vi "working.vi"() -> ()   [LabVIEW 2017]
uses:
  <vilib>/myRIO/Instrument Drivers/Onboard IO/DIO/typedefs/DIO Reference.ctl
  <vilib>/myRIO/Common/Instrument Driver Framework/Utilities/typedefs/myRIO Generic Hardware Reference.ctl
  <vilib>/myRIO/Common/Instrument Driver Framework/Utilities/typedefs/Hardware Version Enum.ctl
  <vilib>/myRIO/Common/Instrument Driver Framework/Utilities/typedefs/myRIO v1.0 Reference.ctl
  <vilib>/myRIO/Common/Instrument Driver Framework/Utilities/typedefs/Generic FPGA Reference.ctl
  <vilib>/myRIO/Common/Instrument Driver Framework/myRIO v1.0/DIO/typedefs/DIO Channels List.ctl
  <vilib>/myRIO/Common/Instrument Driver Framework/myRIO v1.0/DIO/typedefs/DIO Channels Enum.ctl
  <vilib>/userdefined/High Color/nirio_resource_hc.ctl
  <vilib>/myRIO/Common/Instrument Driver Framework/Utilities/vis/Is FPGA Ref Available.vi
  <vilib>/myRIO/Common/Instrument Driver Framework/myRIO v1.0/DIO/vis/myRIO v1.1 Open DIO.vi
  <vilib>/myRIO/Instrument Drivers/Onboard IO/DIO/vis/Write.vi
  <vilib>/myRIO/Common/Instrument Driver Framework/Utilities/vis/Validate Channels.vi
  <vilib>/myRIO/Common/Instrument Driver Framework/myRIO v1.0/DIO/vis/myRIO v1.0 Reserve DIO.vi
  <vilib>/myRIO/Common/Instrument Driver Framework/myRIO v1.0/Resource Manager/vis/myRIO v1.0 Reserve Channel List.vi
  <vilib>/myRIO/Common/Instrument Driver Framework/myRIO v1.0/DIO/vis/myRIO v1.0 Build MUX Configuration DIO.vi
  <vilib>/myRIO/Common/Instrument Driver Framework/myRIO v1.0/Resource Manager/vis/myRIO v1.0 Reserve Channel.vi
  <vilib>/myRIO/Common/Instrument Driver Framework/myRIO v1.0/Resource Manager/vis/myRIO v1.0 Unreserve Channel.vi
  <vilib>/myRIO/Common/Instrument Driver Framework/myRIO v1.0/Resource Manager/vis/myRIO v1.0 Create Configuration List.vi
  <vilib>/myRIO/Common/Instrument Driver Framework/myRIO v1.0/Resource Manager/vis/myRIO v1.0 Build Mutex Name.vi
  <vilib>/Utility/VariantDataType/GetNumericInfo.vi
  <vilib>/Utility/error.llb/Error Cluster From Error Code.vi
  <vilib>/myRIO/Common/Instrument Driver Framework/myRIO v1.0/myRIO v1.1 Open.vi
  <vilib>/myRIO/Common/Instrument Driver Framework/Utilities/vis/IO Manager.vi
  <vilib>/myRIO/Common/Instrument Driver Framework/Utilities/vis/Configuration Manager.vi
  <vilib>/myRIO/Common/Instrument Driver Framework/myRIO v1.0/Resource Manager/vis/myRIO v1.0 Configure IO.vi
  <vilib>/myRIO/Common/Instrument Driver Framework/myRIO v1.0/myRIO v1.0 Close.vi
  <vilib>/myRIO/Common/Instrument Driver Framework/myRIO v1.0/DIO/vis/myRIO v1.0 Write DIO.vi
  <vilib>/myRIO/Express VI/Onboard Devices/LED/LED Express VI.xnode
  <vilib>/myRIO/Instrument Drivers/Onboard IO/DIO/vis/myRIO DIO Open.xnode
  <vilib>/myRIO/Express VI/Onboard IO/DO/DO Express VI.xnode
  <vilib>/myRIO/Instrument Drivers/Onboard IO/DIO/DIO.lvlib
panel:
  out "Numeric 2":i32
  in  "Array 0-4":i32[](array[numeric])
  out "Numeric":i32
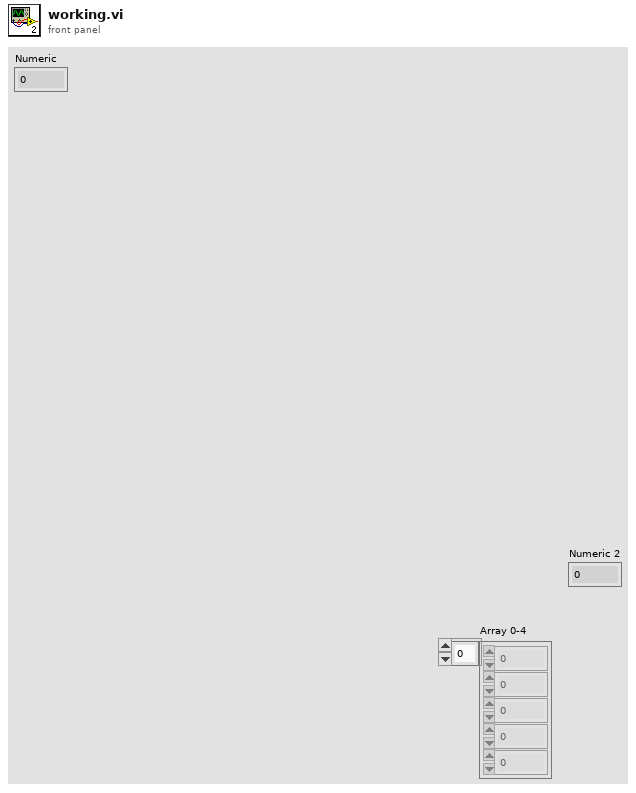
[diagram p1: front panel]
types:
  T1 = typedef "DIO.lvlib/DIO Reference.ctl" = cluster{"myRIO Reference":T2, "DIO Channels List":T6}
  T2 = typedef "myRIO Generic Hardware Reference.ctl" = cluster{"myRIO Model":T3, "myRIO Hardware Reference":T4}
  T3 = typedef "Hardware Version Enum.ctl" = enum16{"Unknown", "myRIO-1900", "myRIO-1950", "roboRIO", "NI ELVIS RIO CM"}
  T4 = typedef "myRIO v1.0 Reference.ctl" = cluster{"Generic FPGA Reference":T5, "Allow multiple opens":bool}
  T5 = typedef "Generic FPGA Reference.ctl" = refnum<k20>
  T6 = typedef "DIO Channels List.ctl" = T7[]
  T7 = typedef "DIO Channels Enum.ctl" = enum16{"Not Connected", "C/DIO0", "C/DIO1", "C/DIO2", "C/DIO3", "C/DIO4", "C/DIO5", "C/DIO6", "C/DIO7", "A/DIO0", "A/DIO1", "A/DIO2", "A/DIO3", "A/DIO4", "A/DIO5", "A/DIO6", "A/DIO7", "A/DIO8", "A/DIO9", "A/DIO10", "A/DIO11", "A/DIO12", "A/DIO13", "A/DIO14", "A/DIO15", "B/DIO0", "B/DIO1", "B/DIO2", "B/DIO3", "B/DIO4", "B/DIO5", "B/DIO6", "B/DIO7", "B/DIO8", "B/DIO9", "B/DIO10", "B/DIO11", "B/DIO12", "B/DIO13", "B/DIO14", "B/DIO15", "LED0", "LED1", "LED2", "LED3", "Button0", "DIO/DIO0", "DIO/DIO1", "DIO/DIO2", "DIO/DIO3", "DIO/DIO4", "DIO/DIO5", "DIO/DIO6", "DIO/DIO7", "DIO/DIO8", "DIO/DIO9", "SPI/CS0", "SPI/CS1", "SPI/CS2", "SPI/CS3", "LED RADIO (Green)", "LED RADIO (Red)", "LED COMM (Green)", "LED COMM (Red)", "LED MODE (Green)", "LED MODE (Red)"}
  T8 = typedef "nirio_resource_hc.ctl" = tag
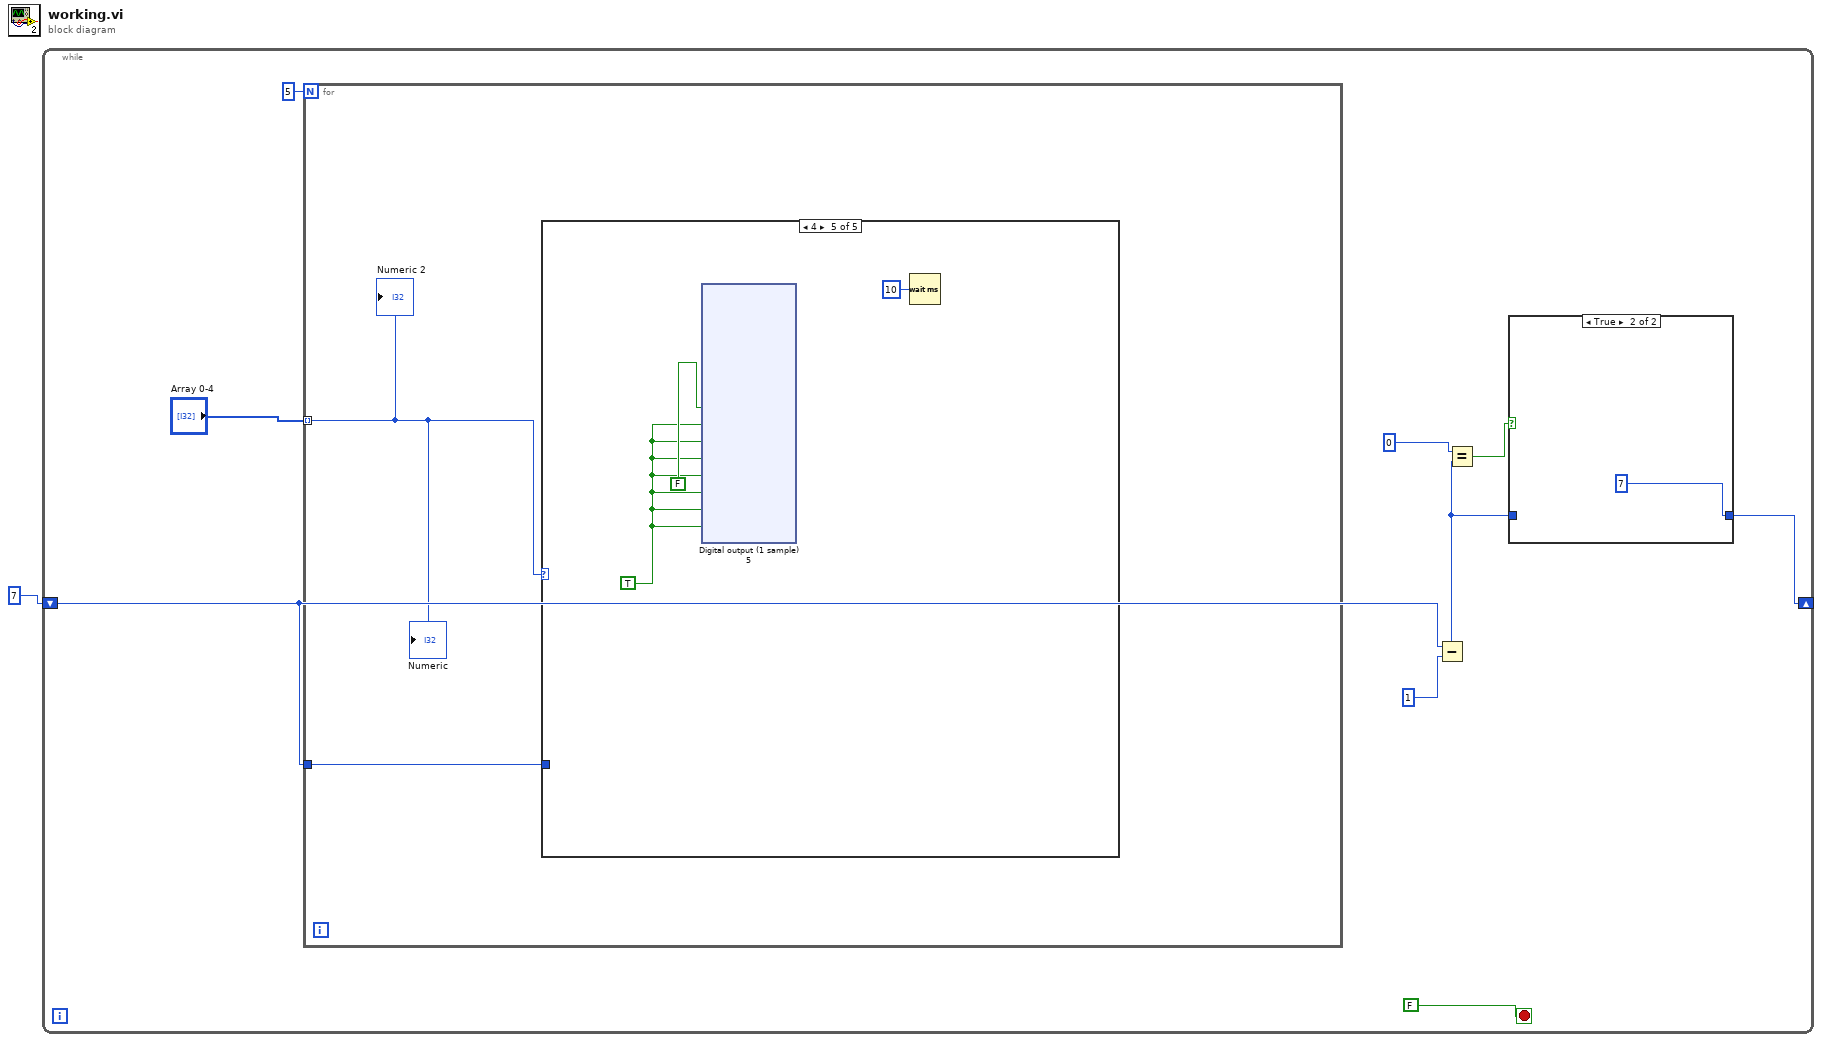
[diagram p0: block diagram]
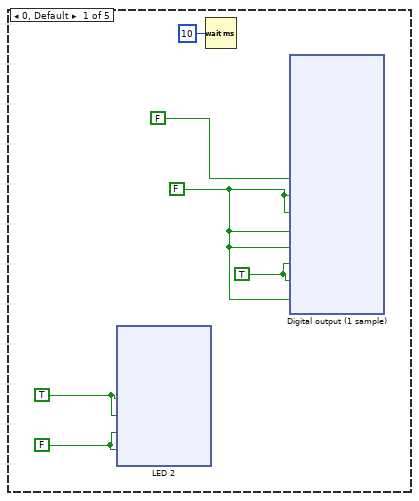
[diagram p3: hidden frame]
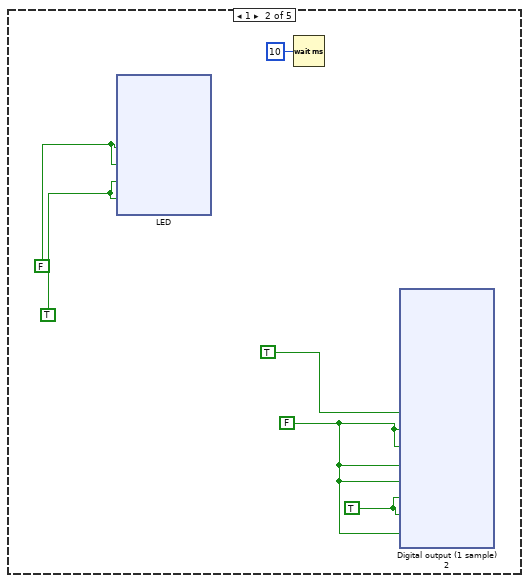
[diagram p4: hidden frame]
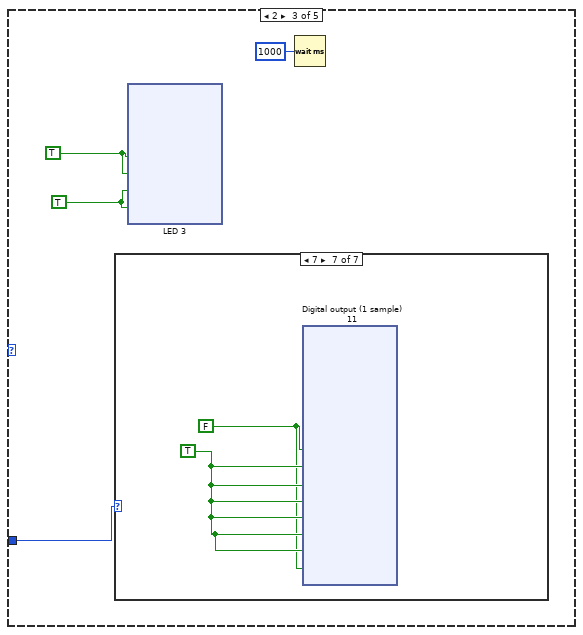
[diagram p5: hidden frame]
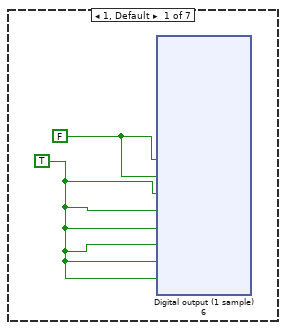
[diagram p6: hidden frame]
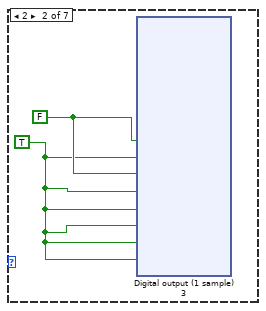
[diagram p7: hidden frame]
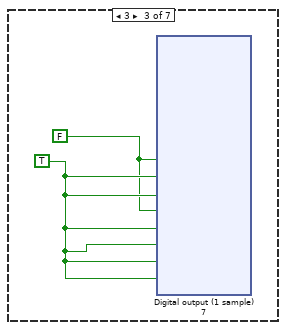
[diagram p8: hidden frame]
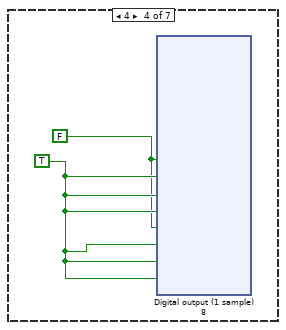
[diagram p9: hidden frame]
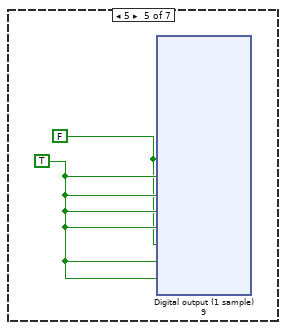
[diagram p10: hidden frame]
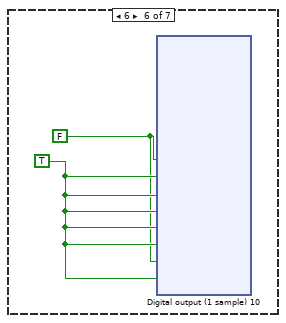
[diagram p11: hidden frame]
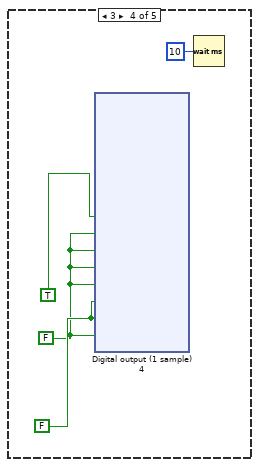
[diagram p12: hidden frame]
diagram:
  n1 = while {
    shift-right: [w2] -> _
    shift-left: 7 -> [w7]
    stop <- FALSE stop-if-true
    n2 = for {
      N: 5 -> [_]
      tunnel: "Array 0-4" -> [w14] mode=indexing
      tunnel: w7 -> [w13]
      n3 = case shown="4" w14 {
        tunnel: w13 -> [_ _ w188 _ _]
        frame 0, Default {
          w16 = TRUE
          w17 = FALSE
          w19 = FALSE
          w20 = TRUE
          n4 = xnode "LED 2"("LED0"=w20, "LED1"=w20, "LED2"=w19, "LED3"=w19) -> ()  [unwired: 1 in, 1 out]
          n5 = Wait (ms)(milliseconds to wait=u32 10) -> ()  [unwired: 1 out]
          n6 = xnode "Digital output (1 sample)"("A/DIO7 (Pin 25)"=FALSE, "A/DIO0 (Pin 11)"=w17, "A/DIO1 (Pin 13)"=w17, "A/DIO2 (Pin 15)"=w17, "A/DIO3 (Pin 17)"=w17, "A/DIO4 (Pin 19)"=w16, "A/DIO5 (Pin 21)"=w16, "A/DIO6 (Pin 23)"=w17) -> ()  [unwired: 1 in, 1 out]
        }
        frame 1 {
          w102 = TRUE
          w103 = FALSE
          w105 = TRUE
          w106 = FALSE
          n7 = xnode "LED"("LED0"=w106, "LED1"=w106, "LED2"=w105, "LED3"=w105) -> ()  [unwired: 1 in, 1 out]
          n8 = Wait (ms)(milliseconds to wait=u32 10) -> ()  [unwired: 1 out]
          n9 = xnode "Digital output (1 sample) 2"("A/DIO7 (Pin 25)"=TRUE, "A/DIO0 (Pin 11)"=w103, "A/DIO1 (Pin 13)"=w103, "A/DIO2 (Pin 15)"=w103, "A/DIO3 (Pin 17)"=w103, "A/DIO4 (Pin 19)"=w102, "A/DIO5 (Pin 21)"=w102, "A/DIO6 (Pin 23)"=w103) -> ()  [unwired: 1 in, 1 out]
        }
        frame 2 {
          w189 = TRUE
          w190 = TRUE
          n10 = case shown="7" w188 {
            frame 1, Default {
              w191 = FALSE
              w192 = TRUE
              n11 = xnode "Digital output (1 sample) 6"("A/DIO7 (Pin 25)"=w191, "A/DIO0 (Pin 11)"=w191, "A/DIO1 (Pin 13)"=w192, "A/DIO2 (Pin 15)"=w192, "A/DIO3 (Pin 17)"=w192, "A/DIO4 (Pin 19)"=w192, "A/DIO5 (Pin 21)"=w192, "A/DIO6 (Pin 23)"=w192) -> ()  [unwired: 1 in, 1 out]
            }
            frame 2 {
              w236 = FALSE
              w235 = TRUE
              n12 = xnode "Digital output (1 sample) 3"("A/DIO7 (Pin 25)"=w236, "A/DIO0 (Pin 11)"=w235, "A/DIO1 (Pin 13)"=w236, "A/DIO2 (Pin 15)"=w235, "A/DIO3 (Pin 17)"=w235, "A/DIO4 (Pin 19)"=w235, "A/DIO5 (Pin 21)"=w235, "A/DIO6 (Pin 23)"=w235) -> ()  [unwired: 1 in, 1 out]
            }
            frame 3 {
              w279 = FALSE
              w280 = TRUE
              n13 = xnode "Digital output (1 sample) 7"("A/DIO7 (Pin 25)"=w279, "A/DIO0 (Pin 11)"=w280, "A/DIO1 (Pin 13)"=w280, "A/DIO2 (Pin 15)"=w279, "A/DIO3 (Pin 17)"=w280, "A/DIO4 (Pin 19)"=w280, "A/DIO5 (Pin 21)"=w280, "A/DIO6 (Pin 23)"=w280) -> ()  [unwired: 1 in, 1 out]
            }
            frame 4 {
              w323 = FALSE
              w324 = TRUE
              n14 = xnode "Digital output (1 sample) 8"("A/DIO7 (Pin 25)"=w323, "A/DIO0 (Pin 11)"=w324, "A/DIO1 (Pin 13)"=w324, "A/DIO2 (Pin 15)"=w324, "A/DIO3 (Pin 17)"=w323, "A/DIO4 (Pin 19)"=w324, "A/DIO5 (Pin 21)"=w324, "A/DIO6 (Pin 23)"=w324) -> ()  [unwired: 1 in, 1 out]
            }
            frame 5 {
              w367 = FALSE
              w368 = TRUE
              n15 = xnode "Digital output (1 sample) 9"("A/DIO7 (Pin 25)"=w367, "A/DIO0 (Pin 11)"=w368, "A/DIO1 (Pin 13)"=w368, "A/DIO2 (Pin 15)"=w368, "A/DIO3 (Pin 17)"=w368, "A/DIO4 (Pin 19)"=w367, "A/DIO5 (Pin 21)"=w368, "A/DIO6 (Pin 23)"=w368) -> ()  [unwired: 1 in, 1 out]
            }
            frame 6 {
              w411 = FALSE
              w412 = TRUE
              n16 = xnode "Digital output (1 sample) 10"("A/DIO7 (Pin 25)"=w411, "A/DIO0 (Pin 11)"=w412, "A/DIO1 (Pin 13)"=w412, "A/DIO2 (Pin 15)"=w412, "A/DIO3 (Pin 17)"=w412, "A/DIO4 (Pin 19)"=w412, "A/DIO5 (Pin 21)"=w411, "A/DIO6 (Pin 23)"=w412) -> ()  [unwired: 1 in, 1 out]
            }
            frame 7 {
              w455 = FALSE
              w456 = TRUE
              n17 = xnode "Digital output (1 sample) 11"("A/DIO7 (Pin 25)"=w455, "A/DIO0 (Pin 11)"=w456, "A/DIO1 (Pin 13)"=w456, "A/DIO2 (Pin 15)"=w456, "A/DIO3 (Pin 17)"=w456, "A/DIO4 (Pin 19)"=w456, "A/DIO5 (Pin 21)"=w456, "A/DIO6 (Pin 23)"=w455) -> ()  [unwired: 1 in, 1 out]
            }
          }
          n18 = xnode "LED 3"("LED0"=w190, "LED1"=w190, "LED2"=w189, "LED3"=w189) -> ()  [unwired: 1 in, 1 out]
          n19 = Wait (ms)(milliseconds to wait=u32 1000) -> ()  [unwired: 1 out]
        }
        frame 3 {
          w540 = FALSE ("A/DIO6 (Pin 23)")
          w539 = FALSE
          n20 = xnode "Digital output (1 sample) 4"("A/DIO7 (Pin 25)"=TRUE, "A/DIO0 (Pin 11)"=w539, "A/DIO1 (Pin 13)"=w539, "A/DIO2 (Pin 15)"=w539, "A/DIO3 (Pin 17)"=w539, "A/DIO4 (Pin 19)"=w540, "A/DIO5 (Pin 21)"=w540, "A/DIO6 (Pin 23)"=w539) -> ()  [unwired: 1 in, 1 out]
          n21 = Wait (ms)(milliseconds to wait=u32 10) -> ()  [unwired: 1 out]
        }
        frame 4 {
          w584 = TRUE
          n22 = xnode "Digital output (1 sample) 5"("A/DIO7 (Pin 25)"=FALSE, "A/DIO0 (Pin 11)"=w584, "A/DIO1 (Pin 13)"=w584, "A/DIO2 (Pin 15)"=w584, "A/DIO3 (Pin 17)"=w584, "A/DIO4 (Pin 19)"=w584, "A/DIO5 (Pin 21)"=w584, "A/DIO6 (Pin 23)"=w584) -> ()  [unwired: 1 in, 1 out]
          n23 = Wait (ms)(milliseconds to wait=u32 10) -> ()  [unwired: 1 out]
        }
      }
      "Numeric" <- w14
      "Numeric 2" <- w14
    }
    n24 = Subtract(x=w7, y=1) -> (x-y=w3:i32)
    n25 = Equal?(x=0, y=w3) -> (x = y?=w4:bool)
    n26 = case shown="True" w4 {
      tunnel: w3 -> [w11 _]
      tunnel: [w11 7] -> w2
      frame False {
      }
      frame True {
      }
    }
  }
